vi "DSBSC2.vi"() -> ()   [LabVIEW 2013]
uses:
  <vilib>/express/express analysis/Spectral/Block/exnSpectralBlock spectral measurements RMS poly.vi
  <vilib>/express/express analysis/Spectral/Block/exnSpectralBlock spectral measurements RMS DDT.vi
  <vilib>/express/express analysis/Spectral/XNode/ExpressSpectralMeasurementsBlockNode.xnode
panel:
  out "Waveform Graph 3":dynamicdata(graph)
  out "Waveform Graph 2":dynamicdata(graph)
  out "Waveform Graph":dynamicdata(graph)
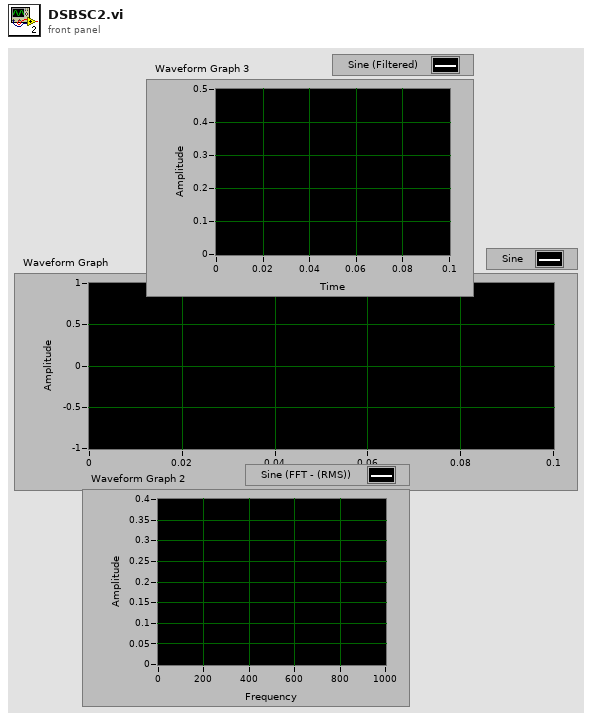
[diagram p1: front panel]
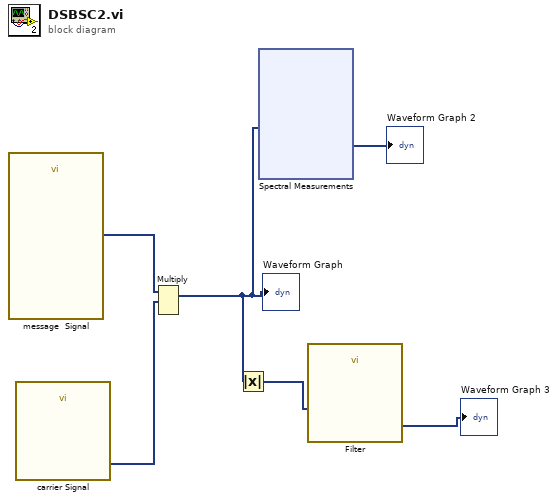
[diagram p0: block diagram]
diagram:
  n1 = call "message  Signal"() -> ("Sine"=w6:dynamicdata)  [unwired: 14 in, 1 out]
  n2 = call "carrier Signal"() -> ("Sine"=w5:dynamicdata)  [unwired: 14 in, 1 out]
  n3 = Multiply(1:w5, 2:w6) -> (0:w3:dynamicdata)  [unwired: 1 in, 1 out]
  "Waveform Graph" <- w3
  n4 = Absolute Value(x=w3) -> (abs(x)=w2:dynamicdata)
  n5 = xnode "Spectral Measurements"("Signals"=w3) -> ("FFT - (RMS)"=→"Waveform Graph 2":dynamicdata)  [unwired: 1 in, 2 out]
  n6 = call "Filter"("Signal"=w2) -> ("Filtered Signal"=→"Waveform Graph 3":dynamicdata)  [unwired: 9 in, 1 out]
